vi "Attenuator Initialize Test.vi"(0 "Instruments to Use":T8, 5 "Seq Count":u32, 9 "Test Parameters In":T9={"Stimulus"={"ATT Stimulus"={"Normalize"=TRUE, "Value (dB)"=0.0}, "VNA Stimulus"={"Use Instrument Settings"=FALSE, "Blank Frequencies"=FALSE, "Sweep Type"=enum."Linear", "Sweep"={"Fstart"=500.0, "Fstop"=1500.0, "Units"=enum."MHz", "Points"=201}, "Power (dBm)"=999.0, "IFBW (Hz)"=-1.0, "Sweep Time (s)"=-1.0, "Calibration"={"State"=FALSE, "String"=""}}}, "Measurement"={"Step (dB)"=enum."0.25", "Start (dB)"=0.0, "Stop (dB)"=31.75}, "Limit"={"Maximum Error"=0.3}, "Normalization"={"Normalized?"=FALSE, "Normalization Values (dB)"=[]}} {"Stimulus"."VNA Stimulus"."Sweep Time (s)" format="%.3g"}, 11 "error in (no error)":errorcluster) -> (4 "Instrument IDs":T6, 6 "Next Action":string, 10 "Test Parameters Out":T9={"Stimulus"={"ATT Stimulus"={"Normalize"=TRUE, "Value (dB)"=0.0}, "VNA Stimulus"={"Use Instrument Settings"=FALSE, "Blank Frequencies"=FALSE, "Sweep Type"=enum."Linear", "Sweep"={"Fstart"=500.0, "Fstop"=1500.0, "Units"=enum."MHz", "Points"=201}, "Power (dBm)"=999.0, "IFBW (Hz)"=-1.0, "Sweep Time (s)"=-1.0, "Calibration"={"State"=FALSE, "String"=""}}}, "Measurement"={"Step (dB)"=enum."0.25", "Start (dB)"=0.0, "Stop (dB)"=31.75}, "Limit"={"Maximum Error"=0.3}, "Normalization"={"Normalized?"=FALSE, "Normalization Values (dB)"=[]}} {"Stimulus"."VNA Stimulus"."Sweep Time (s)" format="%.3g"}, 12 "Calibration":T1, 14 "Driver Refs":T2, 15 "error out":errorcluster {"code" format="%.0x"})   [LabVIEW 2011]
uses:
  TypeDefs/Attenuator Test Parameters.ctl
  TypeDefs/Attenuator Stimulus Parameters.ctl
  TypeDefs/Attenuator ATT Stimulus.ctl
  TypeDefs/Attenuator VNA Stimulus.ctl
  S Parameter/TypeDefs/SP Frequency Units.ctl
  TypeDefs/Attenuator VNA Calibration State.ctl
  TypeDefs/Attenuator Measurement Cluster.ctl
  TypeDefs/Attenuator Limit.ctl
  TypeDefs/Attenuator Calibration State.ctl
  server/database/Stations/Instruments/Instrument Record.ctl
  TypeDefs/Attenuator Driver Refs.ctl
  drivers/ATT/ATT Driver Ref.ctl
  drivers/VNA/VNA Driver Ref.ctl
  drivers/SNA/SNA Driver Ref.ctl
  drivers/ATT/ATT Command.ctl
  S Parameter/TypeDefs/SP Miscellaneous Parameters.ctl
panel:
  in  "Timing Metrics In":string
  in  "Parent VI Refnum":refnum<vi>
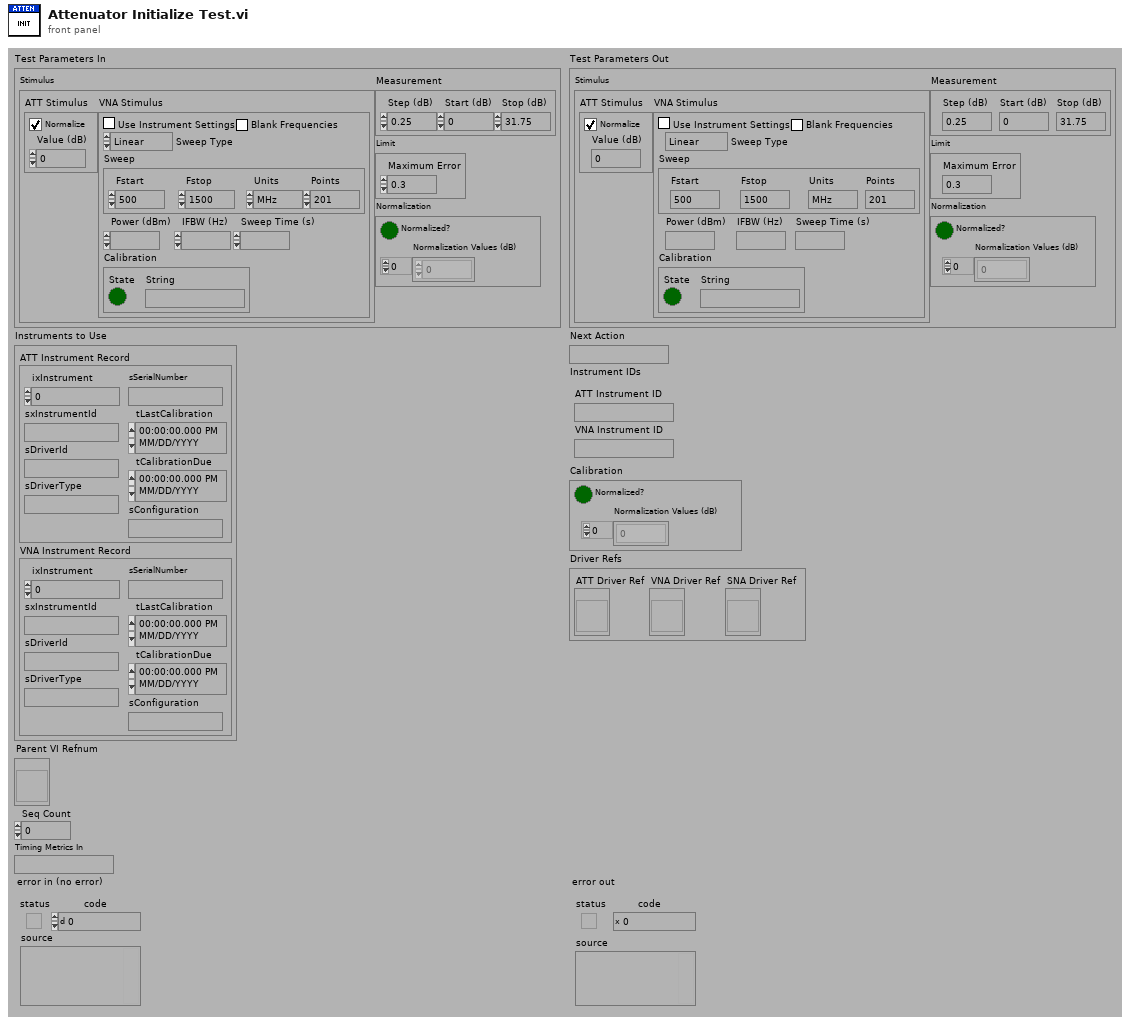
[diagram p1: front panel]
types:
  T1 = typedef "Attenuator Calibration State.ctl" = cluster{"Normalized?":bool, "Normalization Values (dB)":dbl[]}
  T2 = typedef "Attenuator Driver Refs.ctl" = cluster{"ATT Driver Ref":T3, "VNA Driver Ref":T4, "SNA Driver Ref":T5}
  T3 = typedef "ATT Driver Ref.ctl" = refnum<vi>
  T4 = typedef "VNA Driver Ref.ctl" = refnum<vi>
  T5 = typedef "SNA Driver Ref.ctl" = refnum<vi>
  T6 = cluster{"ATT Instrument ID":string, "VNA Instrument ID":string}
  T7 = typedef "Instrument Record.ctl" = cluster{"ixInstrument":i32, "sxInstrumentId":string, "sDriverId":string, "sDriverType":string, "sSerialNumber":string, "tLastCalibration":timestamp, "tCalibrationDue":timestamp, "sConfiguration":string}
  T8 = cluster{"ATT Instrument Record":T7, "VNA Instrument Record":T7}
  T9 = typedef "Attenuator Test Parameters.ctl" = cluster{"Stimulus":T10, "Measurement":T15, "Limit":T16, "Normalization":T1}
  T10 = typedef "Attenuator Stimulus Parameters.ctl" = cluster{"ATT Stimulus":T11, "VNA Stimulus":T12}
  T11 = typedef "Attenuator ATT Stimulus.ctl" = cluster{"Normalize":bool, "Value (dB)":dbl}
  T12 = typedef "Attenuator VNA Stimulus.ctl" = cluster{"Use Instrument Settings":bool, "Blank Frequencies":bool, "Sweep Type":enum32{"Linear", "Logarithmic", "List", "Power", "CW"}, "Sweep":cluster{"Fstart":dbl, "Fstop":dbl, "Units":T13, "Points":i32}, "Power (dBm)":dbl, "IFBW (Hz)":dbl, "Sweep Time (s)":dbl, "Calibration":T14}
  T13 = typedef "SP Frequency Units.ctl" = enum16{"Hz", "kHz", "MHz", "GHz", "Points"}
  T14 = typedef "Attenuator VNA Calibration State.ctl" = cluster{"State":bool, "String":string}
  T15 = typedef "Attenuator Measurement Cluster.ctl" = cluster{"Step (dB)":enum16{"0.25", "0.50", "1.00"}, "Start (dB)":dbl, "Stop (dB)":dbl}
  T16 = typedef "Attenuator Limit.ctl" = cluster{"Maximum Error":dbl}
  T17 = typedef "SP Miscellaneous Parameters.ctl" = cluster{"Formatted Data":bool, "Auto Select":bool, "Seq Count":u32}
  T18 = typedef "ATT Command.ctl" = enum16{"LOAD", "INITIALIZE", "PRESET", "SET STIMULUS", "GET STIMULUS", "GET CALIBRATION", "CALIBRATE", "GET INFO", "RELEASE", "UNLOAD"}
  T19 = cluster{"ATT Flat Output":string, "Instrument ID":string}
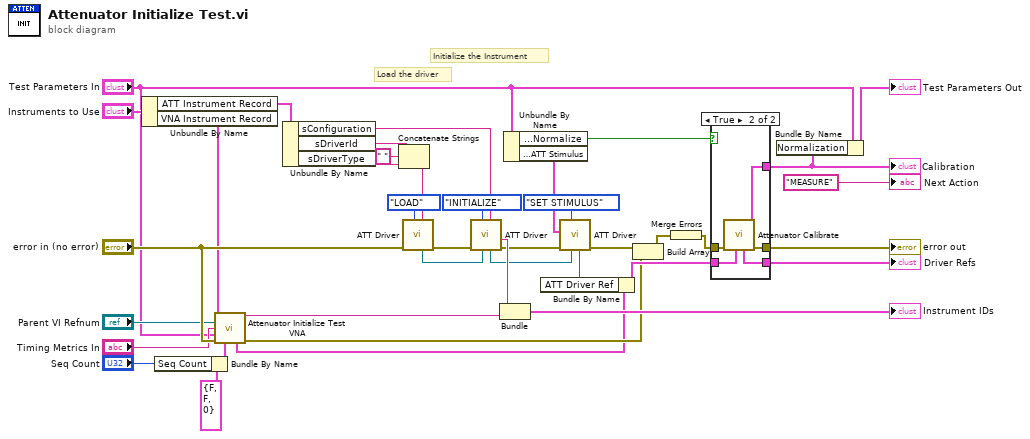
[diagram p0: block diagram]
diagram:
  # "Initialize the Instrument"
  # "Load the driver"
  n1 = Unbundle By Name("Instruments to Use") -> ("ATT Instrument Record"=w23:T7, "VNA Instrument Record"=w15:T7)
  n2 = Bundle By Name(cluster=T17 {"Formatted Data"=FALSE, "Auto Select"=FALSE, "Seq Count"=0} ("Miscellaneous Parameters"), "Seq Count"="Seq Count") -> (w3:T17)
  n3 = call "Attenuator Initialize Test VNA.vi"("Instrument Record"=w15, "Parent VI Refnum"="Parent VI Refnum", "Timing Metrics In"="Timing Metrics In", "Test Parameters In"="Test Parameters In", "error in (no error)"="error in (no error)", "Miscellaneous Parameters"=w3) -> ("Instrument ID"=w10:string, "Driver Ref"=w9:T2, "error out"=w11:errorcluster)  [unwired: 4 in, 3 out]
  n4 = Unbundle By Name(w23) -> ("sConfiguration"=w27:string, "sDriverId"=w26:string, "sDriverType"=w30:string)
  n5 = Concatenate Strings(w26, " " ("string"), w30) -> (w29:string)
  n6 = call "ATT Driver.vi"("ATT Configuration (\"\")"=w29, "ATT Command"=ATT_Command."LOAD", "error in (no error)"="error in (no error)") -> ("error out"=w31:errorcluster, "dup Drv Refnum"=w22:T3)  [unwired: 5 in, 2 out]
  n7 = call "ATT Driver.vi"("ATT Configuration (\"\")"=w27, "Drv Refnum"=w22, "ATT Command"=ATT_Command."INITIALIZE", "error in (no error)"=w31) -> ("error out"=w5:errorcluster, "ATT Flat Output"=w24:string, "dup Drv Refnum"=w6:T3)  [unwired: 4 in, 1 out]
  n8 = Bundle("ATT Flat Output"=w24, "Instrument ID"=w10) -> (→"Instrument IDs":T19)  [unwired: 1 out]
  n9 = Unbundle By Name("Test Parameters In") -> ("Stimulus.ATT Stimulus.Normalize"=w7:bool, "Stimulus.ATT Stimulus"=w8:T11)
  n10 = call "ATT Driver.vi"("Drv Refnum"=w6, "ATT Command"=ATT_Command."SET STIMULUS", "error in (no error)"=w5, "ATT Value In"=w8) -> ("error out"=w21:errorcluster, "dup Drv Refnum"=w18:T3)  [unwired: 4 in, 2 out]
  n11 = Bundle By Name(cluster=w9, "ATT Driver Ref"=w18) -> (w17:T2)
  n12 = Build Array(w21, w11) -> (w25:errorcluster[])
  n13 = Merge Errors(w25) -> (w20:errorcluster)
  n14 = case shown="True" w7 {
    tunnel: w20 -> [w41 w46]
    tunnel: [w41 w44] -> w36
    tunnel: w17 -> [w40 w45]
    tunnel: [w40 w43] -> w39
    tunnel: [_ w42] -> w35
    frame False {
    }
    frame True {
      n15 = call "Attenuator Calibrate.vi"("Driver Refs"=w45, "error in (no error)"=w46) -> ("error out"=w44:errorcluster, "Calibration Out"=w42:T1, "Driver Refs Out"=w43:T2)  [unwired: 7 in]
    }
  }
  "error out" <- w36
  "Driver Refs" <- w39
  "Calibration" <- w35
  n16 = Bundle By Name(cluster="Test Parameters In", "Normalization"=w35) -> (→"Test Parameters Out":T9)
  "Next Action" <- "MEASURE" ("Next Action")
